vi "交替采样泵.vi"(4 "error in (no error)":errorcluster, 7 "队列":refnum<queue>) -> (0 "error out":errorcluster, 3 "队列输出":refnum<queue>)   [LabVIEW 2016, in "PLC.lvlib"]
uses:
  PLC.lvlib
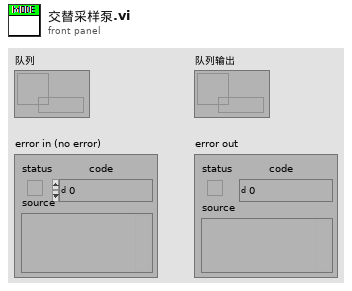
[diagram p1: front panel]
types:
  T1 = cluster{"命令":string, "数据":cluster{"starting address":u16, "holding register values":u16[]}}
  T2 = typedef "LVDateTimeRec.ctl" = cluster{"秒数的小数部分":dbl, "秒":i32, "分":i32, "时":i32, "日":i32, "月":i32, "年":i32, "天数（周）":i32, "天数（年）":i32, "DST":i32}
  T3 = typedef "采配水类型.ctl" = enum16{"V1", "V2", "V3", "V4", "室内V1", "室内V2", "固定站V1", "固定站V2", "浮船V1", "浮船V2"}
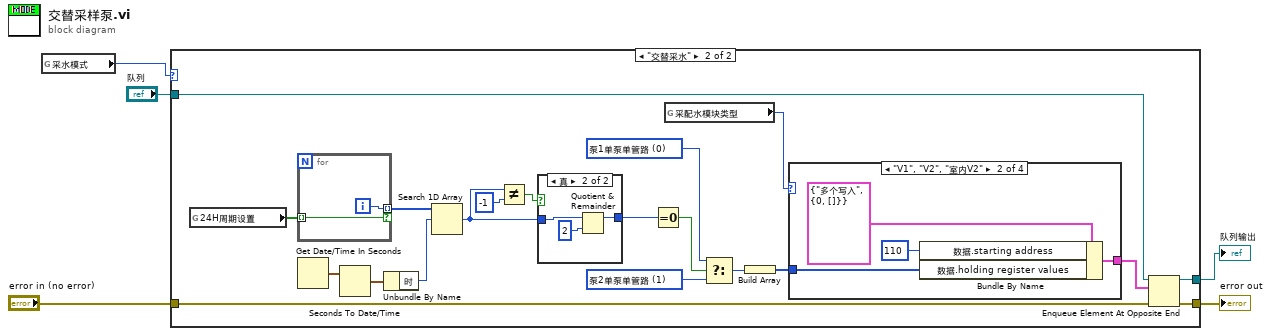
[diagram p0: block diagram]
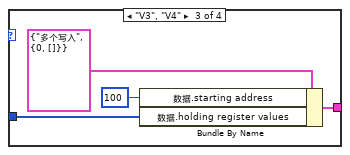
[diagram p5: hidden frame]
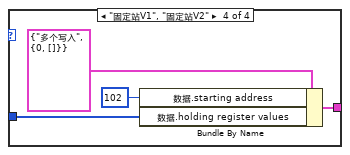
[diagram p6: hidden frame]
diagram:
  n1 = global read "系统设置全局变量.vi" "采水模式"() -> (w5:enum16{"单采水点", "交替采水"})
  n2 = case shown="\"交替采水\"" w5 {
    tunnel: "队列" -> [w7 w11]
    tunnel: "error in (no error)" -> [w6 w10]
    tunnel: [w6 w9] -> w2
    tunnel: [w7 w8] -> w1
    frame "单采水点", Default {
    }
    frame "交替采水" {
      w20 = u16 1 items=["泵1单泵单管路", "泵2单泵单管路"] ("潜水泵工作模式")
      w19 = u16 0 items=["泵1单泵单管路", "泵2单泵单管路"] ("潜水泵工作模式")
      n3 = global read "系统设置全局变量.vi" "24H周期设置"() -> (w13:bool[])
      n4 = for {
        tunnel: w13 -> [w31] mode=indexing
        tunnel: [w32] -> w14 mode=indexing if=w31
        i -> [w32]
      }
      n5 = Get Date/Time In Seconds() -> (seconds since 1Jan1904=w24:timestamp)
      n6 = Seconds To Date/Time(time stamp (now)=w24) -> (date time rec=w15:T2)  [unwired: 1 in]
      n7 = Unbundle By Name(w15) -> ("时"=w16:i32)
      n8 = Search 1D Array(1D array=w14, element=w16) -> (index of element=w21:i32)  [unwired: 1 in]
      n9 = Not Equal?(x=w21, y=-1) -> (x != y?=w23:bool)
      n10 = case shown="真" w23 {
        tunnel: [_ w29] -> w17
        tunnel: w21 -> [_ w28]
        frame False {
        }
        frame True {
          n11 = Quotient & Remainder(x=w28, y=2) -> (x-y*floor(x/y)=w29:i32)  [unwired: 1 out]
        }
      }
      n12 = Equal To 0?(x=w17) -> (x = 0?=w18:bool)
      n13 = global read "系统设置全局变量.vi" "采配水模块类型"() -> (w26:T3)
      n14 = Select(t=w19, s=w18, f=w20) -> (s? t:f=w12:u16)
      n15 = Build Array(w12) -> (w25:u16[])
      n16 = case shown="\"V1\", \"V2\", \"室内V2\"" w26 {
        tunnel: [_ w34 w38 w42] -> w27
        tunnel: w25 -> [_ w33 w37 w41]
        frame Default {
        }
        frame "V1", "V2", "室内V2" {
          n17 = Bundle By Name(cluster=T1 {"命令"="多个写入", "数据"={"starting address"=0, "holding register values"=[]}} ("元素"), "数据.starting address"=u16 110, "数据.holding register values"=w33) -> (w34:T1)
        }
        frame "V3", "V4" {
          n18 = Bundle By Name(cluster=T1 {"命令"="多个写入", "数据"={"starting address"=0, "holding register values"=[]}} ("元素"), "数据.starting address"=u16 100, "数据.holding register values"=w37) -> (w38:T1)
        }
        frame "固定站V1", "固定站V2" {
          n19 = Bundle By Name(cluster=T1 {"命令"="多个写入", "数据"={"starting address"=0, "holding register values"=[]}} ("元素"), "数据.starting address"=u16 102, "数据.holding register values"=w41) -> (w42:T1)
        }
      }
      n20 = Enqueue Element At Opposite End(queue=w11, element=w27, error in (no error)=w10) -> (queue out=w8:refnum<queue>, error out=w9:errorcluster)  [unwired: 1 in, 1 out]
    }
  }
  "error out" <- w2
  "队列输出" <- w1
